vi "Elevator Controller.vi"(8 "error in":errorcluster) -> ()   [LabVIEW 2018]
doc: "This VI executes continuously carrying out the current operation and responding to updates or new operations. It will often contain the timing or control code that is difficult to place directly in TeleOp. This VI generally opens all sensors and motors and isolates the rest of the robot code from knowing how the operations are carried out."
uses:
  <vilib>/Rock Robotics/WPI/Framework/Completion Status.ctl
  Elevator Setpoints.ctl
  Elevator Operations.ctl
  Private/Typedef/Elevator Settings.ctl
  <vilib>/Rock Robotics/WPI/ThirdParty/REV Robotics/SPARK MAX/Typedef/Spark MAX Smart Motion Parameters.ctl
  Private/Typedef/Controller Data.ctl
  <vilib>/Rock Robotics/WPI/MotorControl/WPI_MotorControlDeviceRef.ctl
  <vilib>/Rock Robotics/WPI/MotorControl/WPI_MotorControlType.ctl
  <vilib>/Rock Robotics/SystemInterfaces/DIO/FPGA_DIOPWMChannel.ctl
  <vilib>/Rock Robotics/WPI/PWM/WPI_PWMDeadband.ctl
  <vilib>/Rock Robotics/SystemInterfaces/DIO/FPGA_DIOChannel.ctl
  Elevator Telemetry.ctl
  Elevator Published Globals.vi
panel:
  out "PID Chart":T1(graph)={"Sensor Velocity"=-0.0, "Setpoint"=0.33333587646484375, "Sensor Position"=0.42857396602630615, "Applied Output"=-0.0}
  in  "Settings":T2={"min speed"=0.0, "Position Max"=55.0, "gravity"=0.03, "PID Constants"={"P Gain"=5e-05, "I Gain"=0.0, "D Gain"=1e-05, "F Gain"=0.00015, "I Zone"=0.0, "Min Output"=-1.0, "Max Output"=1.0}, "SM Params"={"Max Velocity"=6200.0, "Max Acceleration"=12000.0, "Minimum Velocity Output"=0.0, "Allowed Closed Loop Error"=0.01}} {"gravity" format="%#_13g"; "Position Max" format="%#_13g"; "min speed" format="%#_13g"}
  out "Switches":T4
  in  "Interactive Values":T5={"Operation"=enum."Go to Position", "Setpoint"=0.0, "Duration"=0.0}
  out "Current\nCmd":string="Started at  13:35:19.542\nDefault: Reserve,  S 0.0, D 0.000000"
  in  "Buttons":cluster{"Execute Cmd":bool, "Abort Cmd":bool}
  out "Command Timing":cluster{"Start Time (ms)":u32, "Iterations":i32}={"Start Time (ms)"=878800, "Iterations"=0}
  out "Status":T7
  # "Interactive Command: You may fill in the settings for a command\nand schedule it with the Execute button. You can observe and abort\nany command while fine tuning the code for the controller."
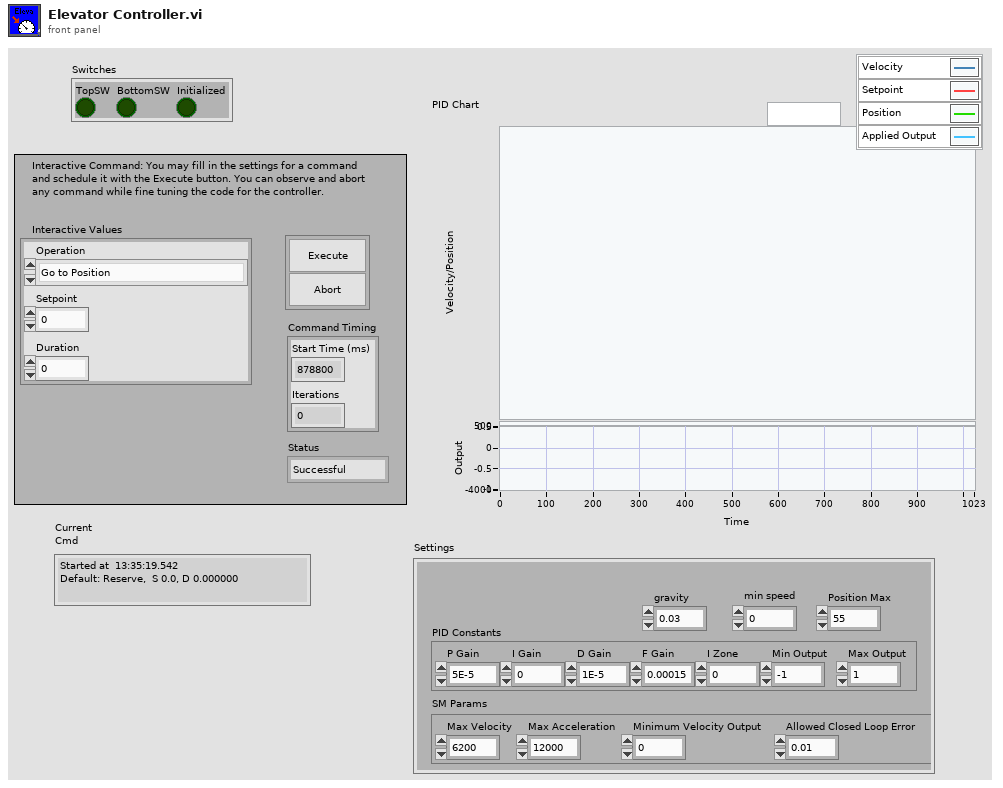
[diagram p1: front panel]
types:
  T1 = cluster{"Sensor Velocity":dbl, "Setpoint":dbl, "Sensor Position":dbl, "Applied Output":dbl}
  T2 = typedef "Elevator Settings.ctl" = cluster{"min speed":dbl, "Position Max":dbl, "gravity":dbl, "PID Constants":cluster{"P Gain":dbl, "I Gain":dbl, "D Gain":dbl, "F Gain":dbl, "I Zone":dbl, "Min Output":dbl, "Max Output":dbl}, "SM Params":T3}
  T3 = typedef "Spark MAX Smart Motion Parameters.ctl" = cluster{"Max Velocity":dbl, "Max Acceleration":dbl, "Minimum Velocity Output":dbl, "Allowed Closed Loop Error":dbl}
  T4 = cluster{"TopSW":bool, "BottomSW":bool, "Initialized":bool}
  T5 = typedef "Elevator Setpoints.ctl" = cluster{"Operation":T6, "Setpoint":dbl, "Duration":dbl}
  T6 = typedef "Elevator Operations.ctl" = enum16{"Reserve", "Read Current", "Immediate", "Stop", "Switch", "Scale", "Home", "Go to Position"}
  T7 = typedef "Completion Status.ctl" = enum16{"Successful", "Aborted", "Incomplete"}
  T8 = typedef "Controller Data.ctl" = cluster{"Setpoint":dbl, "Output":dbl, "DriveMotor1":T9, "Is Done Moving?":bool}
  T9 = typedef "WPI_MotorControlDeviceRef.ctl" = cluster{"DeviceStatus":errorcluster, "Type":T10, "PWM":cluster{"PWM Channel":T11, "DeadBand":T12}, "CAN":cluster{"Device Number":u8, "SetOutput VI Ref":variant, "GetOutput VI Ref":variant, "Enable VI Ref":variant, "Disable VI Ref":variant, "Data":variant}, "Invert":bool, "DIO PWM":cluster{"PWM \"Enable\" Channel":T11, "DIOChannel":T13, "PWM Rate":dbl}}
  T10 = typedef "WPI_MotorControlType.ctl" = enum16{"PWM", "CAN", "DIO PWM"}
  T11 = typedef "FPGA_DIOPWMChannel.ctl" = enum8{"PWM 0", "PWM 1", "PWM 2", "PWM 3", "PWM 4", "PWM 5", "PWM 6", "PWM 7", "PWM 8", "PWM 9", "PWM MXP 0", "PWM MXP 1", "PWM MXP 2", "PWM MXP 3", "PWM MXP 4", "PWM MXP 5", "PWM MXP 6", "PWM MXP 7", "PWM MXP 8", "PWM MXP 9", "Invalid"}
  T12 = typedef "WPI_PWMDeadband.ctl" = cluster{"Name":string, "maxPositivePwm":i32, "minPositivePwm":i32, "centerPwm":i32, "maxNegativePwm":i32, "minNegativePwm":i32, "angularRange":u16}
  T13 = typedef "FPGA_DIOChannel.ctl" = enum8{"DIO 0", "DIO 1", "DIO 2", "DIO 3", "DIO 4", "DIO 5", "DIO 6", "DIO 7", "DIO 8", "DIO 9", "DIO MXP 0", "DIO MXP 1", "DIO MXP 2", "DIO MXP 3", "DIO MXP 4", "DIO MXP 5", "DIO MXP 6", "DIO MXP 7", "DIO MXP 8", "DIO MXP 9", "DIO MXP 10", "DIO MXP 11", "DIO MXP 12", "DIO MXP 13", "DIO MXP 14", "DIO MXP 15", "SPI Port CS1", "SPI Port CS2", "SPI Port CS3", "SPI Port MISO", "SPI Port MOSI", "Invalid"}
  T14 = typedef "Command Status Info.ctl" = cluster{"Name":string, "Status":T7, "notifier out":T15}
  T15 = typedef "Completion Notifier.ctl" = refnum<notifier>
  T16 = cluster{"Current Command":T5, "Command Timing":cluster{"Start Time (ms)":u32, "Iterations":i32}, "Command Arguments":cluster{"Command Info":T14, "Description":string, "Default Command":T5, "queue out":refnum<queue>, "Subsystem Name":string}}
  T17 = typedef "Elevator Telemetry.ctl" = cluster{"Is Moving?":bool, "Setpoint":dbl, "Velocity":dbl, "Position":dbl, "Top Limit":bool, "Bottom Limit":bool, "Applied Output":dbl}
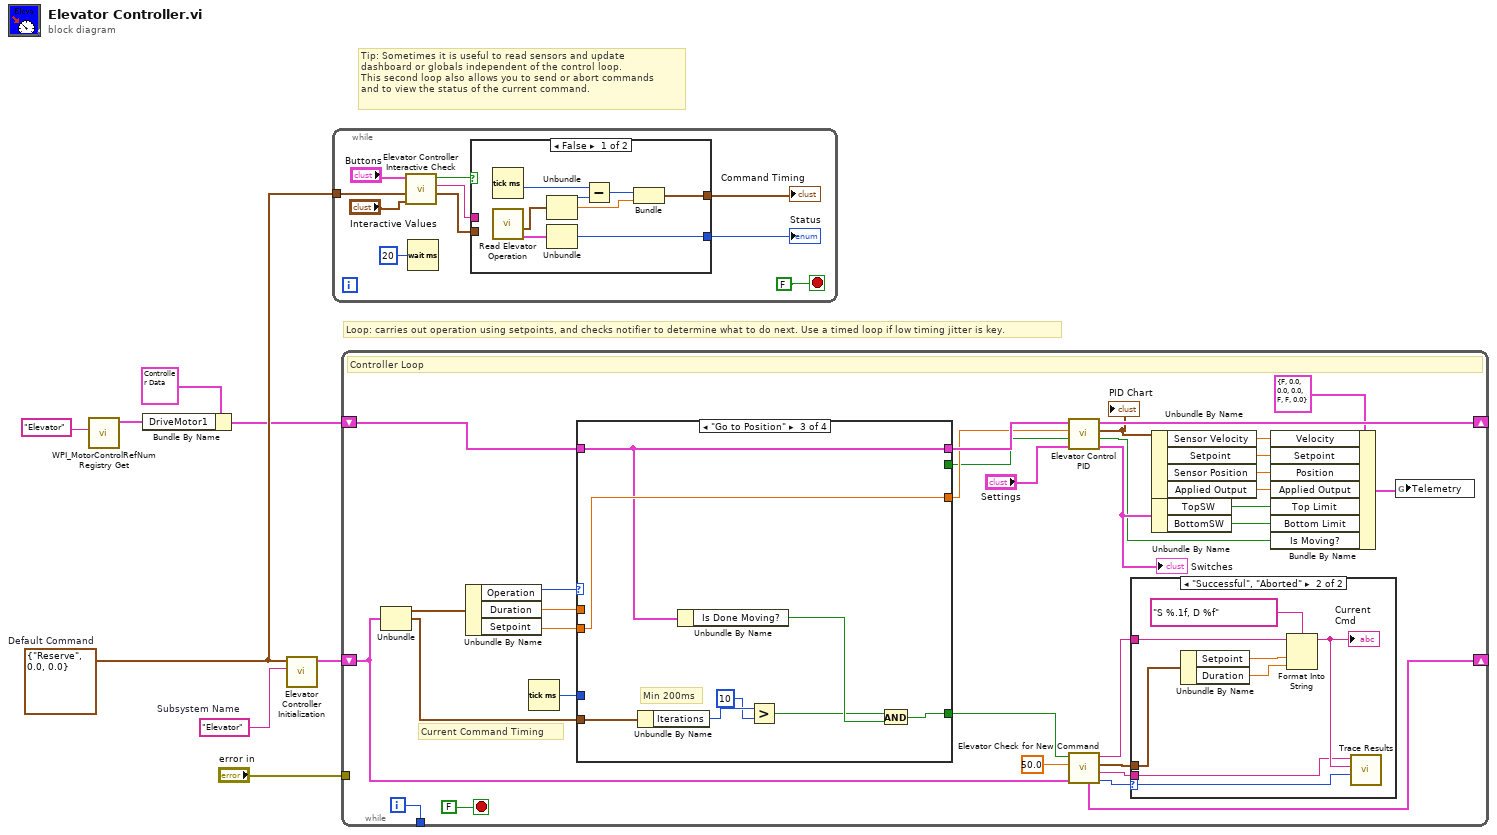
[diagram p0: block diagram]
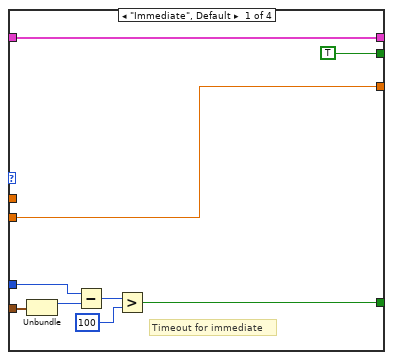
[diagram p2: hidden frame]
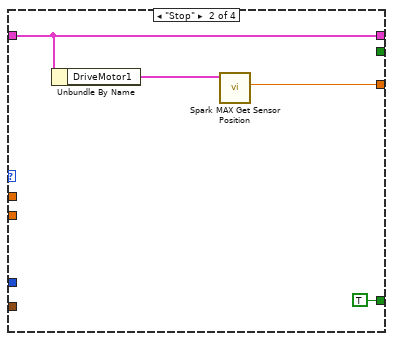
[diagram p3: hidden frame]
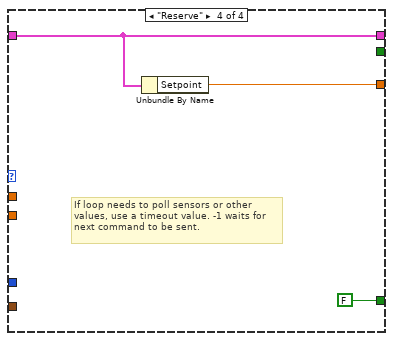
[diagram p4: hidden frame]
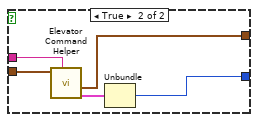
[diagram p6: hidden frame]
diagram:
  w6 = T5 {"Operation"=enum."Reserve", "Setpoint"=0.0, "Duration"=0.0}  # Default Command
  w7 = "Elevator"  # Subsystem Name
  # "Tip: Sometimes it is useful to read sensors and update\ndashboard or globals independent of the control loop.\nThis second loop also allows you to send or abort commands\nand to view the status of the current command."
  # "Loop: carries out operation using setpoints, and checks notifier to determine what to do next. Use a timed loop if low timing jitter is key."
  n1 = call <vilib>:"WPI_MotorControlRefNum Registry Get.vi"("refnum name"="Elevator") -> ("MotorControlDevRef"=w3:T9)  [unwired: 9 in, 1 out]
  n2 = Bundle By Name(cluster=T8 {"Setpoint"=0.0, "Output"=0.0, "DriveMotor1"={"DeviceStatus"={"status"=FALSE, "code"=0, "source"=""}, "Type"=enum."PWM", "PWM"={"PWM Channel"=enum."Invalid", "DeadBand"={"Name"="", "maxPositivePwm"=0, "minPositivePwm"=0, "centerPwm"=0, "maxNegativePwm"=0, "minNegativePwm"=0, "angularRange"=0}}, "CAN"={"Device Number"=0, "SetOutput VI Ref"=variant(enum8{"Percent VBus", "Current", "Speed", "Position", "Voltage"} enum."Percent VBus"), "GetOutput VI Ref"=variant(refnum<k1> refnum), "Enable VI Ref"=variant(dbl 12.0), "Disable VI Ref"=variant(enum8{"Percent VBus", "Speed", "Position", "Slave", "Unchanged / Invalid"} enum."Percent VBus"), "Data"=variant(enum16{"Controller 1"} enum."Controller 1")}, "Invert"=FALSE, "DIO PWM"={"PWM \"Enable\" Channel"=enum."Invalid", "DIOChannel"=enum."Invalid", "PWM Rate"=0.0}}, "Is Done Moving?"=FALSE}, "DriveMotor1"=w3) -> (w2:T8)
  n3 = call "Elevator Controller Initialization.vi"("Subsystem Name"=w7, "Default Command"=w6) -> ("Current Command"=w5:T16)  [unwired: 9 in]
  n4 = while {
    tunnel: w6 -> [w15]
    stop <- FALSE stop-if-true
    n5 = call "Elevator Controller Interactive Check.vi"("Interactive Command in"="Interactive Values", "Default Command"=w15, "Buttons"="Buttons") -> ("Interactive Command out"=w12:T5, "Trace String"=w13:string, "Schedule"=w14:bool)  [unwired: 6 in]
    n6 = Wait (ms)(milliseconds to wait=u32 20) -> ()  [unwired: 1 out]
    n7 = case shown="False" w14 {
      tunnel: [w26 w31] -> w11
      tunnel: w12 -> [_ w29]
      tunnel: [w22 w27] -> w10
      tunnel: w13 -> [_ w30]
      frame False {
        n8 = Tick Count (ms)() -> (millisecond timer value=w21:u32)
        n9 = call "Read Elevator Operation.vi"() -> ("Command Info"=w19:T14, "SubSystem Data"=w20:T5)  [unwired: 9 in, 1 out]
        n10 = Unbundle(w20) -> ("Operation"=w25:T6, "Setpoint"=w23:dbl)  [unwired: 1 out]
        n11 = Unbundle(w19) -> ("Status"=w26:T7)  [unwired: 2 out]
        n12 = Subtract(x=w21, y=w25) -> (x-y=w24:u32)
        n13 = Bundle(w24, "Setpoint"=w23) -> (w22:cluster{u32, "Setpoint":dbl})  [unwired: 1 in]
      }
      frame True {
        n14 = call "Elevator Command Helper.vi"("Description"=w30, "SubSystem Data"=w29) -> ("Command Info Out"=w28:T14, "Command Timing"=w27:cluster{"Start Time (ms)":u32, "Iterations":i32})  [unwired: 7 in, 1 out]
        n15 = Unbundle(w28) -> ("Status"=w31:T7)  [unwired: 2 out]
      }
    }
    "Status" <- w11
    "Command Timing" <- w10
  }
  n16 = while {
    shift-right: [w56] -> _
    shift-left: w5 -> [w50]
    tunnel: [w63] -> _
    tunnel: "error in" -> [_]
    shift-right: [w47] -> _
    shift-left: w2 -> [w49]
    i -> [w63]
    stop <- FALSE stop-if-true
    # "Current Command Timing"
    # "Controller Loop"
    n17 = Unbundle(w50) -> ("Current Command"=w62:T5, "Command Timing"=w58:cluster{"Start Time (ms)":u32, "Iterations":i32})  [unwired: 1 out]
    n18 = Unbundle By Name(w62) -> ("Operation"=w61:T6, "Duration"=w60:dbl, "Setpoint"=w57:dbl)
    n19 = Tick Count (ms)() -> (millisecond timer value=w59:u32)
    n20 = case shown="\"Go to Position\"" w61 {
      tunnel: [w68 TRUE ("ignore previous (F)") w79 FALSE ("ignore previous (F)")] -> w55
      tunnel: w58 -> [w70 _ w82 _]
      tunnel: w60 -> [_ _ _ _]
      tunnel: w59 -> [w69 _ _ _]
      tunnel: w57 -> [w65 _ w85 _]
      tunnel: w49 -> [w67 w77 w84 w87]
      tunnel: [w67 w77 w84 w87] -> w48
      tunnel: [w65 w74 w85 w86] -> w46
      tunnel: [TRUE _ _ _] -> w45
      frame "Immediate", Default {
        # "Timeout for immediate"
        n21 = Unbundle(w70) -> ("Start Time (ms)"=w73:u32)  [unwired: 1 out]
        n22 = Subtract(x=w69, y=w73) -> (x-y=w72:u32)
        n23 = Greater?(x=w72, y=u8 100 ("Left Motor")) -> (0:w68:bool)
      }
      frame "Stop" {
        n24 = Unbundle By Name(w77) -> ("DriveMotor1"=w75:T9)
        n25 = call <vilib>:"Spark MAX Get Sensor Position.vi"("MotorControlDevRef in"=w75) -> ("Sensor Position"=w74:dbl)  [unwired: 7 in, 3 out]
      }
      frame "Go to Position" {
        # "Min 200ms"
        n26 = Unbundle By Name(w82) -> ("Iterations"=w81:i32)
        n27 = Unbundle By Name(w84) -> ("Is Done Moving?"=w83:bool)
        n28 = Greater?(x=w81, y=10 ("x")) -> (0:w78:bool)
        n29 = And(x=w78, y=w83) -> (x .and. y?=w79:bool)
      }
      frame "Reserve" {
        # "If loop needs to poll sensors or other\nvalues, use a timeout value. -1 waits for\nnext command to be sent."
        n30 = Unbundle By Name(w87) -> ("Setpoint"=w86:dbl)
      }
    }
    n31 = call "Elevator Control PID.vi"("Settings"="Settings", "Manual"=w45, "Setpoint"=w46, "Controller In"=w48) -> ("Switches"=w39:T4, "Path is Done?"=w32:bool, "PID Chart"=w40:T1, "Controller out"=w47:T8)  [unwired: 4 in]
    "Switches" <- w39
    "PID Chart" <- w40
    n32 = call "Elevator Check for New Command.vi"("Current Command"=w50, "Wait time (ms)"=50.0, "Finished?"=w55) -> ("Completion"=w51:T7, "Subsystem Name"=w52:string, "Current Command"=w53:T5, "Initial Trace String"=w54:string, "NextCommand"=w56:T16)  [unwired: 4 in]
    n33 = case shown="\"Successful\", \"Aborted\"" w51 {
      selector: w51 -> [_ w89]
      tunnel: w54 -> [_ w93]
      tunnel: w53 -> [_ w94]
      tunnel: w52 -> [_ w90]
      frame "Incomplete", Default {
        # "Continuing current command"
      }
      frame "Successful", "Aborted" {
        # "Report and setup for next command"
        n34 = Unbundle By Name(w94) -> ("Setpoint"=w96:dbl, "Duration"=w91:dbl)
        n35 = Format Into String(format string="S %.1f, D %f", initial string=w93, w96, w91) -> (resulting string=w92:string)  [unwired: 1 in, 1 out]
        "Current\nCmd" <- w92
        n36 = call <vilib>:"Trace Results.vi"("Status of previous command"=w89, "Description"=w92, "Subsystem"=w90) -> ()  [unwired: 9 in]
      }
    }
    n37 = Unbundle By Name(w40) -> ("Sensor Velocity"=w33:dbl, "Setpoint"=w34:dbl, "Sensor Position"=w35:dbl, "Applied Output"=w36:dbl)
    n38 = Unbundle By Name(w39) -> ("TopSW"=w38:bool, "BottomSW"=w37:bool)
    n39 = Bundle By Name(cluster=T17 {"Is Moving?"=FALSE, "Setpoint"=0.0, "Velocity"=0.0, "Position"=0.0, "Top Limit"=FALSE, "Bottom Limit"=FALSE, "Applied Output"=0.0} ("Telemetry"), "Velocity"=w33, "Setpoint"=w34, "Position"=w35, "Applied Output"=w36, "Top Limit"=w38, "Bottom Limit"=w37, "Is Moving?"=w32) -> (w41:T17)
    n40 = global write "Elevator Published Globals.vi" "Telemetry"(w41) -> ()
  }
